vi "CPP_ReflectSingleSided.vi"(1 "DC Present?":bool, 2 "SingleSidedData":dbl[](array[numeric])) -> (0 "DCandReflectedData":dbl[](array[numeric]))   [LabVIEW 2011]
doc: "Reflects single-sided spectral data for use with double-ended (Unshifted) FFTs. Duplicates the last point of the input sequence to ensure correct length."
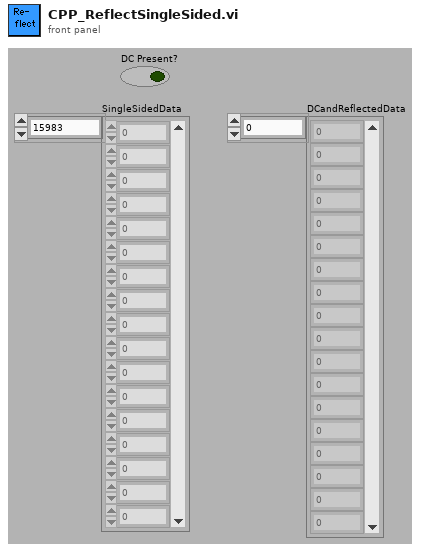
[diagram p1: front panel]
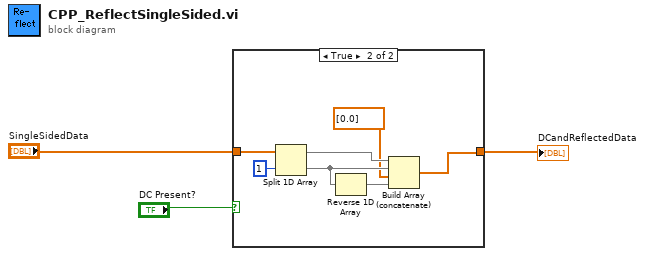
[diagram p0: block diagram]
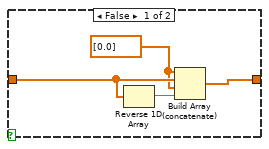
[diagram p2: hidden frame]
diagram:
  n1 = case shown="True" "DC Present?" {
    tunnel: [w7 w12] -> w3
    tunnel: "SingleSidedData" -> [w6 w14]
    frame False {
      w5 = dbl[] [0.0] ("array")
      n2 = Reverse 1D Array(array=w6) -> (reversed array=w4:dbl[])
      n3 = Build Array (concatenate)(w5, w6, w5, w4) -> (w7:dbl[])
    }
    frame True {
      n4 = Split 1D Array(array=w14, index=1) -> (first subarray=w11:dbl[], second subarray=w13:dbl[])
      n5 = Reverse 1D Array(array=w13) -> (reversed array=w9:dbl[])
      n6 = Build Array (concatenate)(w11, w13, dbl[] [0.0] ("array"), w9) -> (w12:dbl[])
    }
  }
  "DCandReflectedData" <- w3
